vi "xijk_create_graphs_excitation.vi"(8 "error in":errorcluster, 11 "Settings":T1={"search parameters"={"Paths"={"Path: Excitation filters"=path "", "Path: Dicroic filters"=path "", "Path: Emission filters"=path "", "Path reget"=path ""}, "table excitation"=[], "table dicroics"=[], "table emission"=[], "Integers"={"Select result number"=1}, "boolean selector array"=[], "table for calculation automagic"=[]}, "output cluster"={"Booleans"={"Unknown detector"=FALSE, "Dual band filters"=FALSE, "Dual emission by cubes"=FALSE, "FRET"=FALSE}, "Integers"={"Light source"=0, "Number of fluorophores"=0, "Wavelength of laser (nm) 1"=0, "Broadness of laser (nm) 1"=0.0, "Wavelength of laser (nm) 2"=0, "Broadness of laser (nm) 2"=0.0, "Template"=1}, "Doubles"={"Molar extinction 1"=1.0, "Molar extinction 2"=1.0, "Quantum efficiency 1"=1.0, "Quantum efficiency 2"=1.0}}, "output cluster 2"={"Excitation filter 1"=path "", "Dichroic filter 1"=path "", "Emission filter 1"=path "", "Excitation filter 2"=path "", "Dichroic filter 2"=path "", "Emission filter 2"=path "", "Extra em filter 1"=path "", "Extra em filter 2"=path "", "Light source file"=path "", "Fluorophore absorption 1"=path "", "Fluorophore emission 1"=path "", "Fluorophore absorption 2"=path "", "Fluorophore emission 2"=path "", "Detector"=path ""}, "cluster de sortie"={"Excitation filter_x"=[], "Excitation filter_y"=[], "Dichroic filter_x"=[], "Dichroic filter_y"=[], "Emission filter_x"=[], "Emission filter_y"=[], "Excitation filter_x 2"=[], "Excitation filter_y 2"=[], "Dichroic filter_x 2"=[], "Dichroic filter_y 2"=[], "Emission filter_x 2"=[], "Emission filter_y 2"=[], "Extra em filter_x 1"=[], "Extra em filter_y 1"=[], "Extra em filter_x 1"=[], "Extra em filter_y 2"=[], "Light source_x"=[], "Light source_y"=[], "Detector_x"=[], "Detector_y"=[], "Fluorophore absorption_x"=[], "Fluorophore absorption_y"=[], "Fluorophore emission_x"=[], "Fluorophore emission_y"=[], "Fluorophore absorption_x 2"=[], "Fluorophore absorption_y 2"=[], "Fluorophore emission_x 2"=[], "Fluorophore emission_y 2"=[], "laser_x"=[], "laser_y"=[], "laser_x 2"=[], "laser_y 2"=[], "quantum efficiency factor 1"=0.0, "quantum efficiency factor 2"=0.0, "lamp scaling factor"=0.0}, "Xijk output cluster"={"Xijk 111"=0.0, "Xijk 112"=0.0, "Xijk 121"=0.0, "Xijk 122"=0.0, "Xijk 211"=0.0, "Xijk 212"=0.0, "Xijk 221"=0.0, "Xijk 222"=0.0, "Eijk 111"=0.0, "Eijk 112"=0.0, "Eijk 121"=0.0, "Eijk 122"=0.0, "Eijk 211"=0.0, "Eijk 212"=0.0, "Eijk 221"=0.0, "Eijk 222"=0.0}, "GUI configuration"={"axes in"={"min x-axis excitation"=300, "max x-axis excitation"=800, "min x-axis emission"=300, "max x-axis emission"=800, "precision of results"=2}, "plot colors in"={"Lanscape Portrait"=FALSE, "Plot logarithmic"=FALSE, "Ex/Em filters double"=FALSE, "Line colors"=[16734569, 56375, 16711916, 5896447, 16448250, 56375]}}, "references"={"Excitation filter 1 ref"=refnum, "Dichroic filter 1 ref"=refnum, "Emission filter 1 ref"=refnum, "Excitation filter 2 ref"=refnum, "Dichroic filter 2 ref"=refnum, "Emission filter 2 ref"=refnum, "Extra em filter 1 ref"=refnum, "Extra em filter 2 ref"=refnum, "Light source file ref"=refnum, "Fluorophore absorption 1 ref"=refnum, "Fluorophore emission 1 ref"=refnum, "Fluorophore absorption 2 ref"=refnum, "Fluorophore emission 2 ref"=refnum, "Detector ref"=refnum}} {"GUI configuration"."axes in"."precision of results" max=8 step=1}) -> (0 "error out":errorcluster, 1 "Filter cube 2 emission":cluster{"Y":dbl[], "Y":dbl[]}[](graph), 2 "Filter cube 1 emission":cluster{"Y":dbl[], "Y":dbl[]}[](graph), 3 "Filter cube 2 excitation":cluster{"Y":dbl[], "Y":dbl[]}[](graph), 5 "Filter cube 1 excitation":cluster{"Y":dbl[], "Y":dbl[]}[](graph))   [LabVIEW 2009]
uses:
  Type Def/settings.ctl
  Type Def/search_parameters.ctl
  Type Def/spectra_parameters.ctl
  Type Def/filepath.ctl
  Type Def/spectrum_table_control.ctl
  Type Def/xijk_cluster.ctl
  Type Def/configuration_cluster.ctl
  Type Def/axis_parameters.ctl
  Type Def/color_parameters.ctl
  Type Def/control_references_cluster.ctl
panel:
  # "Dichroic"
  # "Ex/Em filter"
  # "Fluorophore 1"
  # "Fluorophore 2"
  # "Laser /\nextra Em filter"
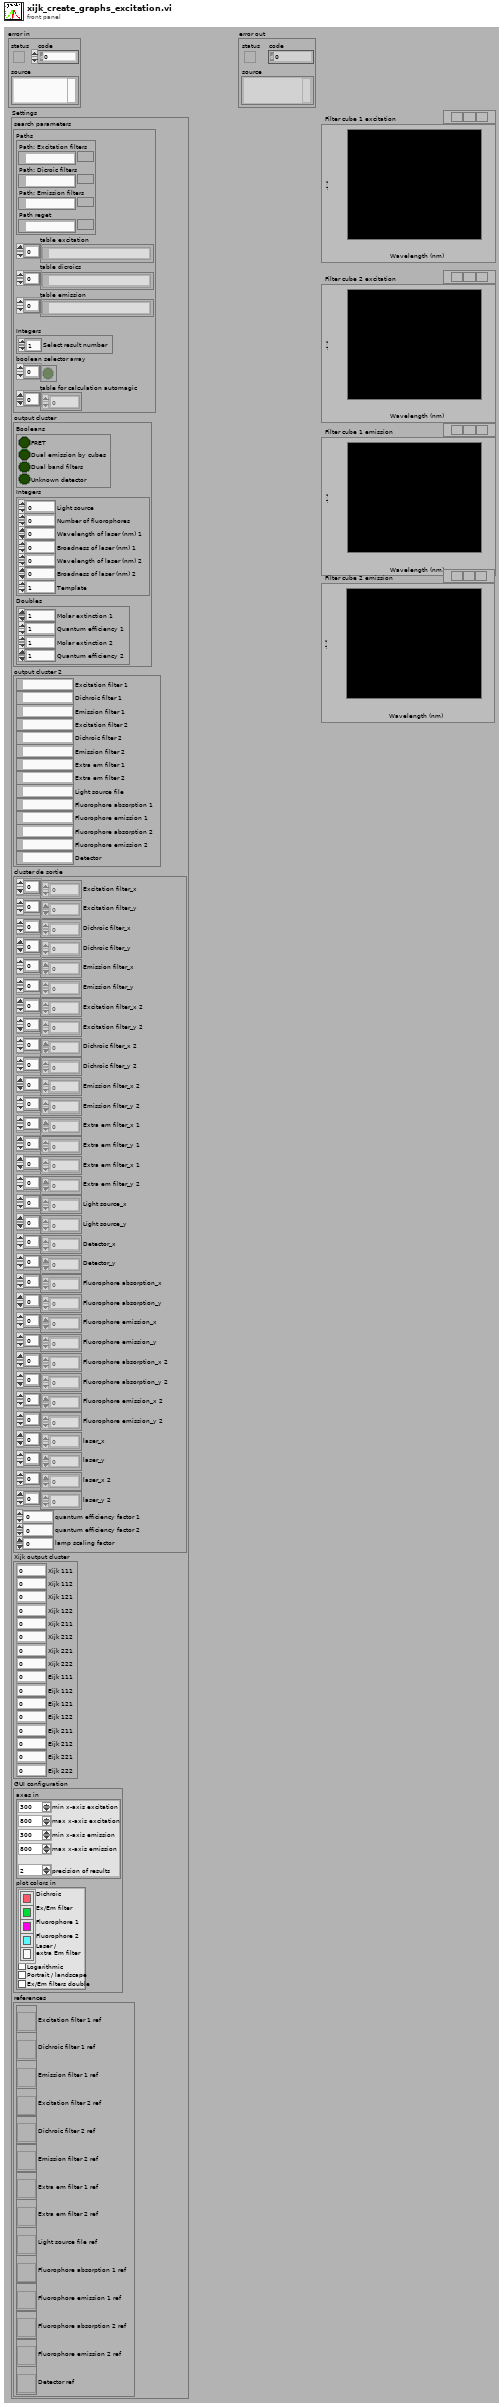
[diagram p1: front panel]
types:
  T1 = typedef "settings.ctl" = cluster{"search parameters":T2, "output cluster":T3, "output cluster 2":T4, "cluster de sortie":T5, "Xijk output cluster":T6, "GUI configuration":T7, "references":T10}
  T2 = typedef "search_parameters.ctl" = cluster{"Paths":cluster{"Path: Excitation filters":path, "Path: Dicroic filters":path, "Path: Emission filters":path, "Path reget":path}, "table excitation":path[], "table dicroics":path[], "table emission":path[], "Integers":cluster{"Select result number":u32}, "boolean selector array":bool[], "table for calculation automagic":i32[]}
  T3 = typedef "spectra_parameters.ctl" = cluster{"Booleans":cluster{"Unknown detector":bool, "Dual band filters":bool, "Dual emission by cubes":bool, "FRET":bool}, "Integers":cluster{"Light source":u16, "Number of fluorophores":u16, "Wavelength of laser (nm) 1":u16, "Broadness of laser (nm) 1":sgl, "Wavelength of laser (nm) 2":u16, "Broadness of laser (nm) 2":sgl, "Template":u16}, "Doubles":cluster{"Molar extinction 1":sgl, "Molar extinction 2":sgl, "Quantum efficiency 1":sgl, "Quantum efficiency 2":sgl}}
  T4 = typedef "filepath.ctl" = cluster{"Excitation filter 1":path, "Dichroic filter 1":path, "Emission filter 1":path, "Excitation filter 2":path, "Dichroic filter 2":path, "Emission filter 2":path, "Extra em filter 1":path, "Extra em filter 2":path, "Light source file":path, "Fluorophore absorption 1":path, "Fluorophore emission 1":path, "Fluorophore absorption 2":path, "Fluorophore emission 2":path, "Detector":path}
  T5 = typedef "spectrum_table_control.ctl" = cluster{"Excitation filter_x":i16[], "Excitation filter_y":sgl[], "Dichroic filter_x":i16[], "Dichroic filter_y":sgl[], "Emission filter_x":i16[], "Emission filter_y":sgl[], "Excitation filter_x 2":i16[], "Excitation filter_y 2":sgl[], "Dichroic filter_x 2":i16[], "Dichroic filter_y 2":sgl[], "Emission filter_x 2":i16[], "Emission filter_y 2":sgl[], "Extra em filter_x 1":i16[], "Extra em filter_y 1":sgl[], "Extra em filter_x 1":i16[], "Extra em filter_y 2":sgl[], "Light source_x":i16[], "Light source_y":sgl[], "Detector_x":i16[], "Detector_y":sgl[], "Fluorophore absorption_x":i16[], "Fluorophore absorption_y":sgl[], "Fluorophore emission_x":i16[], "Fluorophore emission_y":sgl[], "Fluorophore absorption_x 2":i16[], "Fluorophore absorption_y 2":sgl[], "Fluorophore emission_x 2":i16[], "Fluorophore emission_y 2":sgl[], "laser_x":i16[], "laser_y":sgl[], "laser_x 2":i16[], "laser_y 2":sgl[], "quantum efficiency factor 1":sgl, "quantum efficiency factor 2":sgl, "lamp scaling factor":sgl}
  T6 = typedef "xijk_cluster.ctl" = cluster{"Xijk 111":sgl, "Xijk 112":sgl, "Xijk 121":sgl, "Xijk 122":sgl, "Xijk 211":sgl, "Xijk 212":sgl, "Xijk 221":sgl, "Xijk 222":sgl, "Eijk 111":sgl, "Eijk 112":sgl, "Eijk 121":sgl, "Eijk 122":sgl, "Eijk 211":sgl, "Eijk 212":sgl, "Eijk 221":sgl, "Eijk 222":sgl}
  T7 = typedef "configuration_cluster.ctl" = cluster{"axes in":T8, "plot colors in":T9}
  T8 = typedef "axis_parameters.ctl" = cluster{"min x-axis excitation":u16, "max x-axis excitation":u16, "min x-axis emission":u16, "max x-axis emission":u16, "precision of results":u8}
  T9 = typedef "color_parameters.ctl" = cluster{"Lanscape Portrait":bool, "Plot logarithmic":bool, "Ex/Em filters double":bool, "Line colors":u32[]}
  T10 = typedef "control_references_cluster.ctl" = cluster{"Excitation filter 1 ref":refnum<vi>, "Dichroic filter 1 ref":refnum<vi>, "Emission filter 1 ref":refnum<vi>, "Excitation filter 2 ref":refnum<vi>, "Dichroic filter 2 ref":refnum<vi>, "Emission filter 2 ref":refnum<vi>, "Extra em filter 1 ref":refnum<vi>, "Extra em filter 2 ref":refnum<vi>, "Light source file ref":refnum<vi>, "Fluorophore absorption 1 ref":refnum<vi>, "Fluorophore emission 1 ref":refnum<vi>, "Fluorophore absorption 2 ref":refnum<vi>, "Fluorophore emission 2 ref":refnum<vi>, "Detector ref":refnum<vi>}
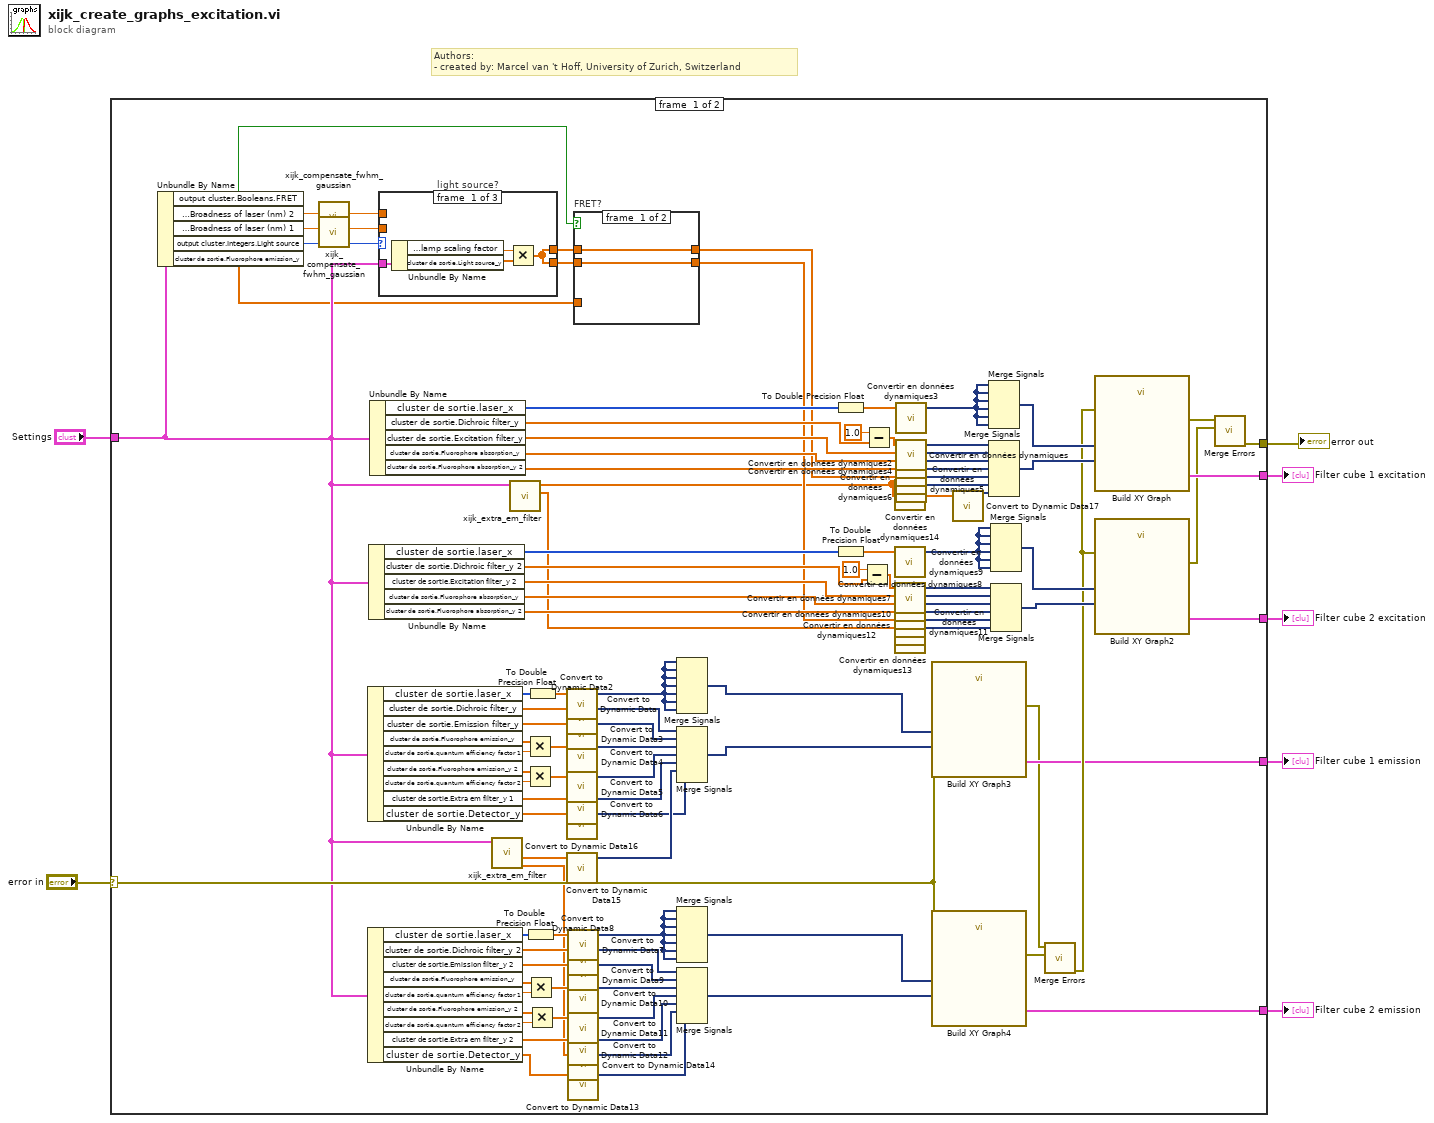
[diagram p0: block diagram]
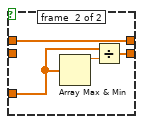
[diagram p2: hidden frame]
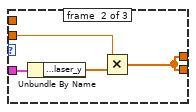
[diagram p3: hidden frame]
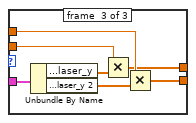
[diagram p4: hidden frame]
diagram:
  # "Authors: \n- created by: Marcel van 't Hoff, University of Zurich, Switzerland"
  n1 = case shown="No Error" "error in" {
    selector: "error in" -> [w36 w135]
    tunnel: [w91 _] -> w7
    tunnel: [w90 _] -> w6
    tunnel: [w75 w135] -> w5
    tunnel: [w34 _] -> w3
    tunnel: [w33 _] -> w2
    tunnel: "Settings" -> [w17 _]
    frame #0 {
      n2 = Unbundle By Name(w17) -> ("output cluster.Booleans.FRET"=w80:bool, "output cluster.Integers.Broadness of laser (nm) 2"=w16:sgl, "output cluster.Integers.Broadness of laser (nm) 1"=w15:sgl, "output cluster.Integers.Light source"=w81:u16, "cluster de sortie.Fluorophore emission_y"=w14:sgl[])
      n3 = call "xijk_compensate_fwhm_gaussian.vi"("FWHM"=w16) -> ("Numeric"=w24:sgl)  [unwired: 10 in]
      n4 = call "xijk_compensate_fwhm_gaussian.vi"("FWHM"=w15) -> ("Numeric"=w25:sgl)  [unwired: 10 in]
      n5 = Unbundle By Name(w17) -> ("cluster de sortie.laser_x"=w37:i16[], "cluster de sortie.Dichroic filter_y"=w38:sgl[], "cluster de sortie.Emission filter_y"=w41:sgl[], "cluster de sortie.Fluorophore emission_y"=w43:sgl[], "cluster de sortie.quantum efficiency factor 1"=w63:sgl, "cluster de sortie.Fluorophore emission_y 2"=w61:sgl[], "cluster de sortie.quantum efficiency factor 2"=w65:sgl, "cluster de sortie.Extra em filter_y 1"=w46:sgl[], "cluster de sortie.Detector_y"=w20:sgl[])
      n6 = Unbundle By Name(w17) -> ("cluster de sortie.laser_x"=w55:i16[], "cluster de sortie.Dichroic filter_y 2"=w56:sgl[], "cluster de sortie.Emission filter_y 2"=w57:sgl[], "cluster de sortie.Fluorophore emission_y"=w71:sgl[], "cluster de sortie.quantum efficiency factor 1"=w67:sgl, "cluster de sortie.Fluorophore emission_y 2"=w69:sgl[], "cluster de sortie.quantum efficiency factor 2"=w68:sgl, "cluster de sortie.Extra em filter_y 2"=w58:sgl[], "cluster de sortie.Detector_y"=w23:sgl[])
      n7 = Unbundle By Name(w17) -> ("cluster de sortie.laser_x"=w106:i16[], "cluster de sortie.Dichroic filter_y 2"=w112:sgl[], "cluster de sortie.Excitation filter_y 2"=w107:sgl[], "cluster de sortie.Fluorophore absorption_y"=w105:sgl[], "cluster de sortie.Fluorophore absorption_y 2"=w104:sgl[])
      n8 = Unbundle By Name(w17) -> ("cluster de sortie.laser_x"=w101:i16[], "cluster de sortie.Dichroic filter_y"=w109:sgl[], "cluster de sortie.Excitation filter_y"=w100:sgl[], "cluster de sortie.Fluorophore absorption_y"=w102:sgl[], "cluster de sortie.Fluorophore absorption_y 2"=w103:sgl[])
      n9 = case "light source?" shown="2" w81 {
        tunnel: w17 -> [w123 w127 w134]
        tunnel: [w120 w124 w129] -> w79
        tunnel: [w120 w124 w128] -> w78
        tunnel: w25 -> [_ w125 w132]
        tunnel: w24 -> [_ _ w130]
        frame #0 {
          n10 = Unbundle By Name(w123) -> ("cluster de sortie.lamp scaling factor"=w122:sgl, "cluster de sortie.Light source_y"=w121:sgl[])
          n11 = Multiply(x=w122, y=w121) -> (x*y=w120:sgl[])
        }
        frame #1 {
          n12 = Unbundle By Name(w127) -> ("cluster de sortie.laser_y"=w126:sgl[])
          n13 = Multiply(x=w125, y=w126) -> (x*y=w124:sgl[])
        }
        frame #2 {
          n14 = Unbundle By Name(w134) -> ("cluster de sortie.laser_y"=w133:sgl[], "cluster de sortie.laser_y 2"=w131:sgl[])
          n15 = Multiply(x=w132, y=w133) -> (x*y=w129:sgl[])
          n16 = Multiply(x=w130, y=w131) -> (x*y=w128:sgl[])
        }
      }
      n17 = call "xijk_extra_em_filter.vi"("Settings"=w17) -> ("Emission filter_y"=w28:sgl[], "Emission filter_y 2"=w29:sgl[])  [unwired: 7 in, 2 out]
      n18 = call "xijk_extra_em_filter.vi"("Settings"=w17) -> ("Excitation filter_y"=w27:sgl[], "Excitation filter_y 2"=w13:sgl[])  [unwired: 7 in, 2 out]
      n19 = Multiply(x=w43, y=w63) -> (x*y=w62:sgl[])
      n20 = Multiply(x=w61, y=w65) -> (x*y=w64:sgl[])
      n21 = To Double Precision Float(number=w55) -> (double precision float=w59:dbl[])
      n22 = Multiply(x=w71, y=w67) -> (x*y=w72:sgl[])
      n23 = Multiply(x=w69, y=w68) -> (x*y=w70:sgl[])
      n24 = To Double Precision Float(number=w37) -> (double precision float=w60:dbl[])
      n25 = call "Convert to Dynamic Data"("Array"=w60) -> ("Dynamic Data Type"=w18:dynamicdata)  [unwired: 3 in]
      n26 = call "Convert to Dynamic Data2"("Array"=w38) -> ("Dynamic Data Type"=w39:dynamicdata)  [unwired: 3 in]
      n27 = call "Convert to Dynamic Data3"("Array"=w41) -> ("Dynamic Data Type"=w42:dynamicdata)  [unwired: 3 in]
      n28 = call "Convert to Dynamic Data4"("Array"=w62) -> ("Dynamic Data Type"=w44:dynamicdata)  [unwired: 3 in]
      n29 = call "Convert to Dynamic Data5"("Array"=w64) -> ("Dynamic Data Type"=w45:dynamicdata)  [unwired: 3 in]
      n30 = call "Convert to Dynamic Data6"("Array"=w46) -> ("Dynamic Data Type"=w47:dynamicdata)  [unwired: 3 in]
      n31 = call "Convert to Dynamic Data16"("Array"=w20) -> ("Dynamic Data Type"=w19:dynamicdata)  [unwired: 3 in]
      n32 = call "Convert to Dynamic Data15"("Array"=w29) -> ("Dynamic Data Type"=w26:dynamicdata)  [unwired: 3 in]
      n33 = call "Convert to Dynamic Data7"("Array"=w59) -> ("Dynamic Data Type"=w21:dynamicdata)  [unwired: 3 in]
      n34 = call "Convert to Dynamic Data8"("Array"=w56) -> ("Dynamic Data Type"=w54:dynamicdata)  [unwired: 3 in]
      n35 = call "Convert to Dynamic Data9"("Array"=w57) -> ("Dynamic Data Type"=w52:dynamicdata)  [unwired: 3 in]
      n36 = call "Convert to Dynamic Data10"("Array"=w72) -> ("Dynamic Data Type"=w51:dynamicdata)  [unwired: 3 in]
      n37 = call "Convert to Dynamic Data11"("Array"=w70) -> ("Dynamic Data Type"=w50:dynamicdata)  [unwired: 3 in]
      n38 = call "Convert to Dynamic Data12"("Array"=w58) -> ("Dynamic Data Type"=w66:dynamicdata)  [unwired: 3 in]
      n39 = call "Convert to Dynamic Data14"("Array"=w28) -> ("Dynamic Data Type"=w32:dynamicdata)  [unwired: 3 in]
      n40 = call "Convert to Dynamic Data13"("Array"=w23) -> ("Dynamic Data Type"=w22:dynamicdata)  [unwired: 3 in]
      n41 = case "FRET?" shown="True" w80 {
        tunnel: [w115 w119] -> w77
        tunnel: w79 -> [w115 w119]
        tunnel: [w114 w117] -> w76
        tunnel: w78 -> [w114 _]
        tunnel: w14 -> [_ w116]
        frame #0 {
        }
        frame #1 {
          n42 = Array Max & Min(array=w116) -> (max value=w118:sgl)  [unwired: 3 out]
          n43 = Divide(x=w116, y=w118) -> (x/y=w117:sgl[])
        }
      }
      n44 = Merge Signals(w18, w18, w18, w18, w18, w18, w18) -> (w48:dynamicdata)
      n45 = Merge Signals(w39, w42, w44, w45, w47, w26, w19) -> (w40:dynamicdata)
      n46 = Merge Signals(w21, w21, w21, w21, w21, w21, w21) -> (w49:dynamicdata)
      n47 = Merge Signals(w54, w52, w51, w50, w66, w32, w22) -> (w53:dynamicdata)
      n48 = To Double Precision Float(number=w101) -> (double precision float=w74:dbl[])
      n49 = To Double Precision Float(number=w106) -> (double precision float=w73:dbl[])
      n50 = Subtract(x=sgl 1.0, y=w112) -> (x-y=w113:sgl[])
      n51 = Subtract(x=sgl 1.0, y=w109) -> (x-y=w110:sgl[])
      n52 = call "Convertir en données dynamiques14"("Array"=w13) -> ("Dynamic Data Type"=w30:dynamicdata)  [unwired: 3 out]
      n53 = call "Convertir en données dynamiques9"("Array"=w73) -> ("Dynamic Data Type"=w89:dynamicdata)  [unwired: 3 out]
      n54 = call "Convertir en données dynamiques7"("Array"=w113) -> ("Dynamic Data Type"=w88:dynamicdata)  [unwired: 3 out]
      n55 = call "Convertir en données dynamiques8"("Array"=w107) -> ("Dynamic Data Type"=w87:dynamicdata)  [unwired: 3 out]
      n56 = call "Convertir en données dynamiques10"("Array"=w105) -> ("Dynamic Data Type"=w86:dynamicdata)  [unwired: 3 out]
      n57 = call "Convertir en données dynamiques11"("Array"=w104) -> ("Dynamic Data Type"=w85:dynamicdata)  [unwired: 3 out]
      n58 = call "Convertir en données dynamiques12"("Array"=w76) -> ("Dynamic Data Type"=w84:dynamicdata)  [unwired: 3 out]
      n59 = call "Convertir en données dynamiques13"("Array"=w27) -> ("Dynamic Data Type"=w31:dynamicdata)  [unwired: 3 out]
      n60 = call "Convertir en données dynamiques3"("Array"=w74) -> ("Dynamic Data Type"=w94:dynamicdata)  [unwired: 3 out]
      n61 = call "Convertir en données dynamiques"("Array"=w110) -> ("Dynamic Data Type"=w99:dynamicdata)  [unwired: 3 out]
      n62 = call "Convertir en données dynamiques2"("Array"=w100) -> ("Dynamic Data Type"=w98:dynamicdata)  [unwired: 3 out]
      n63 = call "Convertir en données dynamiques4"("Array"=w102) -> ("Dynamic Data Type"=w97:dynamicdata)  [unwired: 3 out]
      n64 = call "Convertir en données dynamiques5"("Array"=w103) -> ("Dynamic Data Type"=w96:dynamicdata)  [unwired: 3 out]
      n65 = call "Convertir en données dynamiques6"("Array"=w77) -> ("Dynamic Data Type"=w95:dynamicdata)  [unwired: 3 out]
      n66 = call "Build XY Graph3"("error in (no error)"=w36, "Y Input"=w40, "X Input"=w48) -> ("error out"=w9:errorcluster, "XY Graph"=w34:cluster{"Y":dbl[], "Y":dbl[]}[])  [unwired: 7 in]
      n67 = call "Build XY Graph4"("error in (no error)"=w36, "Y Input"=w53, "X Input"=w49) -> ("error out"=w8:errorcluster, "XY Graph"=w33:cluster{"Y":dbl[], "Y":dbl[]}[])  [unwired: 7 in]
      n68 = call "Convert to Dynamic Data17"("Array"=w13) -> ("Dynamic Data Type"=w12:dynamicdata)  [unwired: 3 in]
      n69 = Merge Signals(w94, w94, w94, w94, w94, w94) -> (w93:dynamicdata)
      n70 = Merge Signals(w99, w98, w97, w96, w95, w30, w12) -> (w92:dynamicdata)
      n71 = Merge Signals(w89, w89, w89, w89, w89, w89) -> (w83:dynamicdata)
      n72 = Merge Signals(w88, w87, w86, w85, w84, w31) -> (w82:dynamicdata)
      n73 = call <vilib>:"Merge Errors.vi"("error in 2 (no error)"=w8, "error in 1 (no error)"=w9) -> ("error out"=w35:errorcluster)  [unwired: 5 in]
      n74 = call "Build XY Graph"("error in (no error)"=w35, "Y Input"=w92, "X Input"=w93) -> ("error out"=w11:errorcluster, "XY Graph"=w91:cluster{"Y":dbl[], "Y":dbl[]}[])  [unwired: 7 in]
      n75 = call "Build XY Graph2"("error in (no error)"=w35, "Y Input"=w82, "X Input"=w83) -> ("error out"=w10:errorcluster, "XY Graph"=w90:cluster{"Y":dbl[], "Y":dbl[]}[])  [unwired: 7 in]
      n76 = call <vilib>:"Merge Errors.vi"("error in 2 (no error)"=w10, "error in 1 (no error)"=w11) -> ("error out"=w75:errorcluster)  [unwired: 5 in]
    }
    frame #1 {
    }
  }
  "Filter cube 2 excitation" <- w6
  "Filter cube 1 excitation" <- w7
  "error out" <- w5
  "Filter cube 1 emission" <- w3
  "Filter cube 2 emission" <- w2
